vi "Write graphs.vi"(8 "error in (no error)":errorcluster, 10 "graphs":refnum<notifier>, 11 "AbstractCollector1D in":refnum<class "AbstractCollector1D.lvclass">) -> (0 "error out":errorcluster, 3 "AbstractCollector1D out":refnum<class "AbstractCollector1D.lvclass">)   [LabVIEW 2014]
uses:
  AbstractCollector1D.lvclass
  Data/Data Abstraction Layer/Data1D/Data1D.lvclass
  Data1D Cluster.ctl
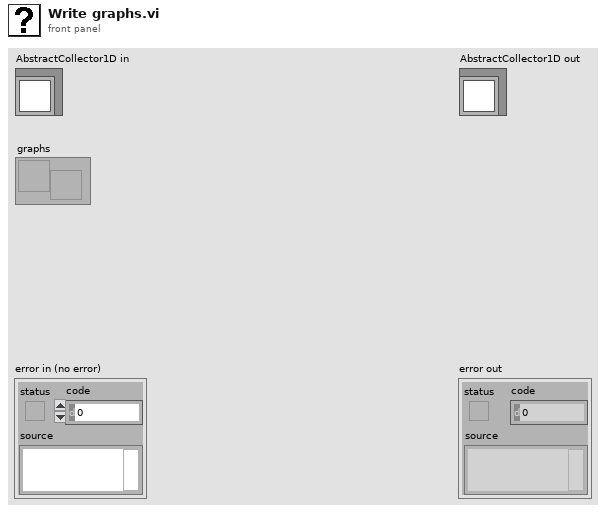
[diagram p1: front panel]
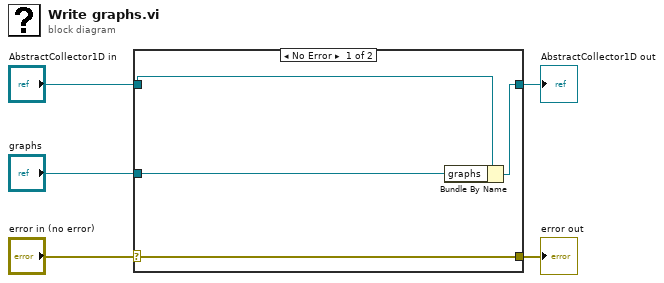
[diagram p0: block diagram]
diagram:
  n1 = case shown="No Error" "error in (no error)" {
    selector: "error in (no error)" -> [w9 w10]
    tunnel: [w9 w10] -> w4
    tunnel: [w7 w11] -> w2
    tunnel: "AbstractCollector1D in" -> [w8 w11]
    tunnel: "graphs" -> [w6 _]
    frame No Error {
      n2 = Bundle By Name(cluster=w8, "graphs"=w6) -> (w7:refnum<class "AbstractCollector1D.lvclass">)
    }
    frame Error {
    }
  }
  "error out" <- w4
  "AbstractCollector1D out" <- w2
